vi "transmit_PN_Using_queue.vi"() -> ()   [LabVIEW 2015]
uses:
  <instrlib>/niUSRP/niUSRP Write Tx Data (CDB).vi
  reference global variable.vi
  reference global variable 2.vi
panel:
  out "coerced gain":dbl format="%#_6f"
  out "coerced carrier frequency":dbl=915000000.0 format="%#_6p"
  out "coerced IQ rate":dbl=1000000.0 format="%#_6p"
  in  "gain":dbl
  in  "carrier frequency":dbl=915000000.0 format="%#_6p"
  in  "fs":dbl=1000000.0 format="%#_6p"
  out "TX2":bool
  out "TX1":bool
  out "Numeric":i32
  out "Samples per period":dbl=127.0
  in  "Samples per chip":i32=1
  in  "Queue length":i32=4
  out "# elements in queue":i32=4
  out "Queue error out":errorcluster
  out "Samples per frame":dbl=1270.0
  out "Array":i32[](array[numeric])=[1, 1, 1, 1, 1, -1, 1, 1, -1, -1, 1, -1, 1, -1, 1, -1, 1, -1, -1, -1, -1, -1, -1, -1, -1, -1, 1, 1, 1, -1, 1, 1, -1, 1, -1, 1, 1, -1, -1, -1, 1, 1, 1, 1, 1, 1, 1, 1, -1, -1, -1, -1, 1, 1, 1, 1, 1, -1, -1, -1, 1, 1, 1, -1, -1, 1, 1, -1, -1, -1, -1, -1, 1, -1, -1, 1, -1, -1, 1, -1, 1, -1, -1, -1, -1, 1, 1, 1, 1, -1, 1, 1, -1, -1, -1, 1, -1, -1, -1, 1, 1, -1, -1, 1, 1, -1, 1, -1, 1, 1, -1, 1, -1, -1, -1, 1, 1, -1, -1, 1, -1, -1, 1, 1, 1, 1, -1]
  in  "PN sequences\n per frame":i32=10
  in  "stop":bool
  out "TX error out":errorcluster
  in  "Device":string="192.168.10.11"
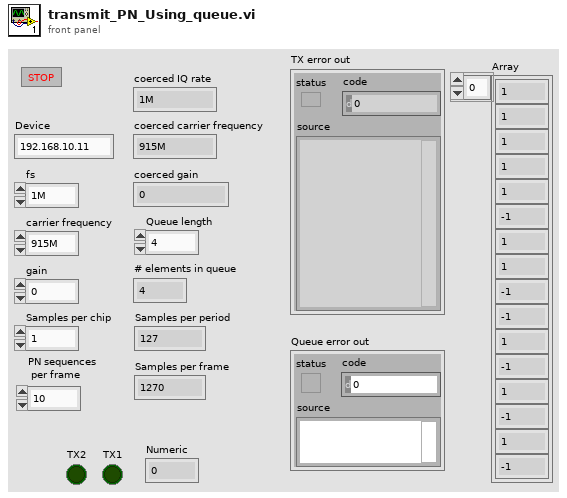
[diagram p1: front panel]
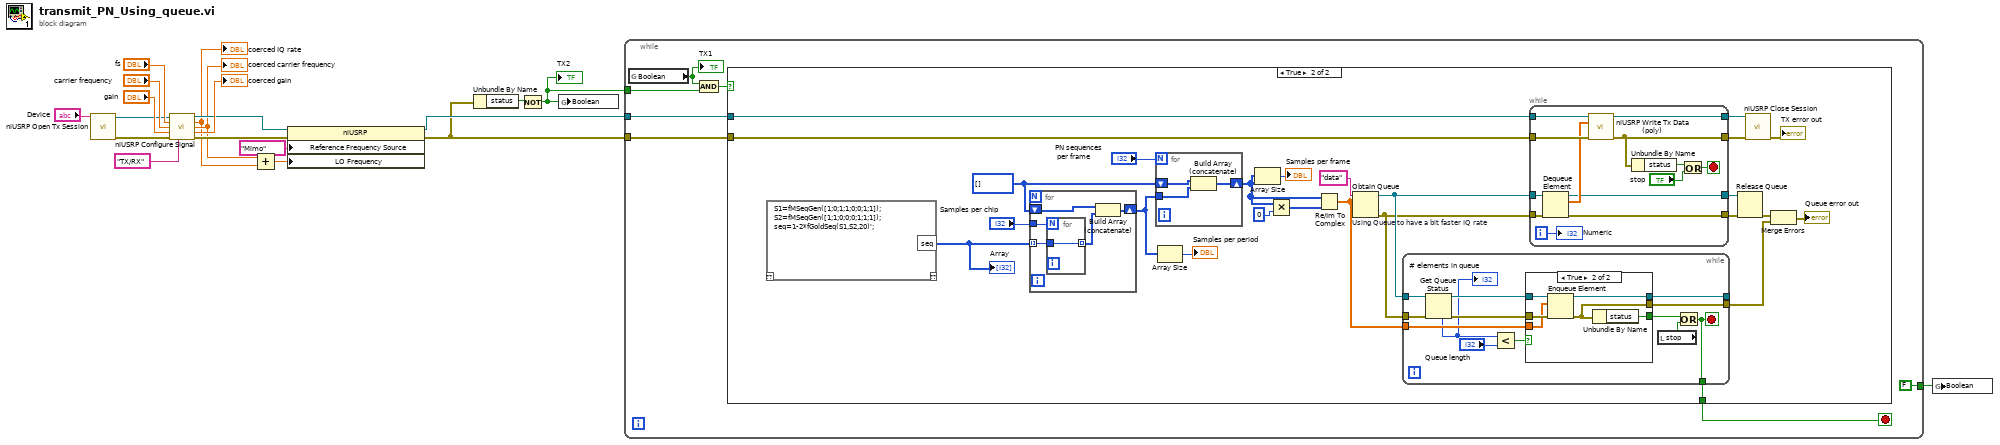
[diagram p0: block diagram]
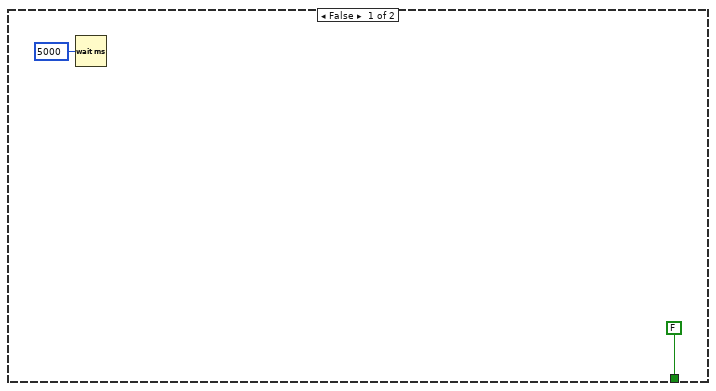
[diagram p2: hidden frame]
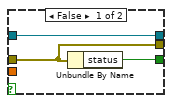
[diagram p3: hidden frame]
diagram:
  n1 = call <instrlib>:"niUSRP Open Tx Session.vi"("device names"="Device") -> ("session handle out"=w11:refnum<k15>, "error out"=w10:errorcluster)  [unwired: 13 in]
  n2 = call <instrlib>:"niUSRP Configure Signal.vi"("session handle"=w11, "IQ rate"="fs", "carrier frequency"="carrier frequency", "gain"="gain", "error in (no error)"=w10, "active antenna"="TX/RX") -> ("session handle out"=w8:refnum<k15>, "coerced IQ rate"=w1:dbl, "coerced carrier frequency"=w2:dbl, "coerced gain"=→"coerced gain":dbl, "error out"=w4:errorcluster)  [unwired: 5 in]
  "coerced IQ rate" <- w1
  "coerced carrier frequency" <- w2
  n3 = Add(x=w2, y=w1) -> (x+y=w5:dbl)
  n4 = property class="niUSRP"(reference=w8, error in=w4, "Reference Frequency Source"="Mimo" ("Clocking and Synchronization:Reference Frequency Source"), "LO Frequency"=w5) -> (reference out=w7:refnum<k15>, error out=w3:errorcluster)
  n5 = Unbundle By Name(w3) -> ("status"=w18:bool)
  n6 = Not(x=w18) -> (.not. x?=w17:bool)
  "TX2" <- w17
  n7 = global write "reference global variable 2.vi" "Boolean"(w17) -> ()
  n8 = while {
    tunnel: w17 -> [w25]
    tunnel: w7 -> [w23]
    tunnel: w3 -> [w22]
    tunnel: [FALSE ("Boolean")] -> w9
    stop <- w21 stop-if-true
    n9 = global read "reference global variable.vi" "Boolean"() -> (w26:bool)
    "TX1" <- w26
    n10 = And(x=w26, y=w25) -> (x .and. y?=w24:bool)
    n11 = case shown="True" w24 {
      tunnel: w23 -> [_ w31]
      tunnel: w22 -> [_ w30]
      tunnel: [FALSE w29] -> w21
      frame False {
        n12 = Wait (ms)(milliseconds to wait=u32 5000) -> ()  [unwired: 1 out]
      }
      frame True {
        w39 = i32[] []
        n13 = mathscript code="S1=fMSeqGen([1;0;1;1;0;0;1;1]);\nS2=fMSeqGen([1;1;0;0;0;1;1;1]);\nseq=1-2*fGoldSeq(S1,S2,20)';"() -> ("seq"=w36:i32[])  [unwired: 1 in, 1 out]
        "Array" <- w36
        n14 = for {
          tunnel: w36 -> [w58] mode=indexing
          tunnel: "Samples per chip" -> [w57]
          shift-right: [w56] -> w37
          shift-left: w39 -> [w54]
          n15 = for {
            N: w57 -> [_]
            tunnel: w58 -> [w59]
            tunnel: [w59] -> w55 mode=indexing
          }
          n16 = Build Array (concatenate)(w54, w55) -> (w56:i32[])
        }
        n17 = for {
          N: "PN sequences\n per frame" -> [_]
          tunnel: w37 -> [w83]
          shift-right: [w82] -> w48
          shift-left: w39 -> [w84]
          n18 = Build Array (concatenate)(w84, w83) -> (w82:i32[])
        }
        n19 = Array Size(array=w37) -> (size(s)=→"Samples per period":i32)
        n20 = Array Size(array=w48) -> (size(s)=→"Samples per frame":i32)
        n21 = Multiply(x=w48, y=0) -> (x*y=w50:i32[])
        n22 = Re/Im To Complex(1:w50, 2:w48) -> (0:w46:cdb[])
        n23 = Obtain Queue "Using Queue to have a bit faster IQ rate"(name (unnamed)="data", element data type=w46) -> (queue out=w45:refnum<queue>, error out=w44:errorcluster)  [unwired: 3 in, 1 out]
        n24 = while {
          tunnel: w46 -> [w68]
          tunnel: w45 -> [w67]
          tunnel: w44 -> [w66]
          tunnel: [w65] -> _
          tunnel: [w64] -> w34
          tunnel: [w60] -> w29
          stop <- w60 stop-if-true
          n25 = Get Queue Status(queue=w67, error in (no error)=w66) -> (queue out=w70:refnum<queue>, error out=w69:errorcluster, # elements in queue=w61:i32)  [unwired: 1 in, 5 out]
          "# elements in queue" <- w61
          n26 = Less?(x=w61, y="Queue length") -> (x < y?=w71:bool)
          n27 = case shown="True" w71 {
            tunnel: w70 -> [w75 w81]
            tunnel: w69 -> [w74 w80]
            tunnel: w68 -> [_ w79]
            tunnel: [w75 w78] -> w65
            tunnel: [w74 w77] -> w64
            tunnel: [w73 w76] -> w63
            frame False {
              n28 = Unbundle By Name(w74) -> ("status"=w73:bool)
            }
            frame True {
              n29 = Enqueue Element(queue=w81, element=w79, error in (no error)=w80) -> (queue out=w78:refnum<queue>, error out=w77:errorcluster)  [unwired: 1 in, 1 out]
              n30 = Unbundle By Name(w77) -> ("status"=w76:bool)
            }
          }
          n31 = local read "stop"() -> (w62:bool)
          n32 = Or(x=w63, y=w62) -> (x .or. y?=w60:bool)
        }
        n33 = while {
          tunnel: w30 -> [w97]
          tunnel: [w96] -> w53
          tunnel: w45 -> [w93]
          tunnel: w44 -> [w92]
          tunnel: [w90] -> w43
          tunnel: [w89] -> w42
          tunnel: w31 -> [w86]
          tunnel: [w85] -> w32
          i -> [w87]
          stop <- w88 stop-if-true
          n34 = Dequeue Element(queue=w93, error in (no error)=w92) -> (queue out=w90:refnum<queue>, element=w91:cdb[], error out=w89:errorcluster)  [unwired: 1 in, 1 out]
          n35 = call-poly <instrlib>:"niUSRP Write Tx Data (poly).vi"("session handle"=w86, "data"=w91, "error in (no error)"=w97) -> ("session handle out"=w85:refnum<k15>, "error out"=w96:errorcluster)  [unwired: 11 in]
          n36 = Unbundle By Name(w96) -> ("status"=w95:bool)
          n37 = Or(x=w95, y="stop") -> (x .or. y?=w88:bool)
          "Numeric" <- w87
        }
        n38 = Release Queue(queue=w43, error in (no error)=w42) -> (error out=w35:errorcluster)  [unwired: 1 in, 2 out]
        n39 = call <instrlib>:"niUSRP Close Session.vi"("session handle"=w32, "error in (no error)"=w53) -> ("error out"=→"TX error out":errorcluster)  [unwired: 13 in]
        n40 = Merge Errors(w35, w34) -> (→"Queue error out":errorcluster)
      }
    }
  }
  n41 = global write "reference global variable 2.vi" "Boolean"(w9) -> ()
